vi "poly_range_DBL.vi"(8 "inclusive (T)":bool=TRUE, 9 "end":dbl, 10 "beginning":dbl) -> (1 "range":dbl[](array[numeric]), 2 "N":i32)   [LabVIEW 2015]
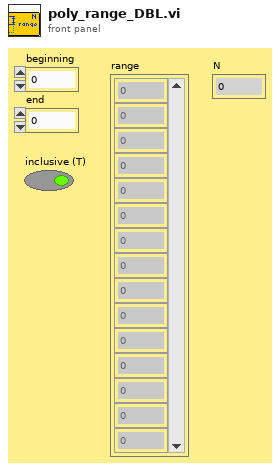
[diagram p1: front panel]
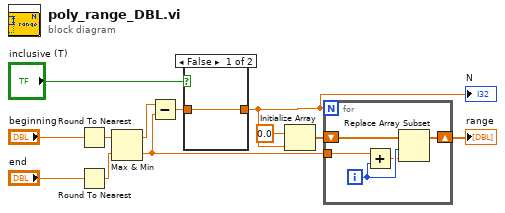
[diagram p0: block diagram]
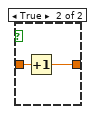
[diagram p2: hidden frame]
diagram:
  n1 = Round To Nearest(number="beginning") -> (nearest integer value=w3:dbl)
  n2 = Round To Nearest(number="end") -> (nearest integer value=w1:dbl)
  n3 = Max & Min(x=w3, y=w1) -> (max(x,y)=w12:dbl, min(x,y)=w9:dbl)
  n4 = Subtract(x=w12, y=w9) -> (x-y=w7:dbl)
  n5 = case shown="False" "inclusive (T)" {
    tunnel: w7 -> [w13 w15]
    tunnel: [w13 w14] -> w6
    frame False {
    }
    frame True {
      n6 = Increment(x=w15) -> (x+1=w14:dbl)
    }
  }
  "N" <- w6
  n7 = Initialize Array(0.0, w6) -> (w10:dbl[])
  n8 = for {
    N: w6 -> [_]
    shift-right: [w16] -> w8
    shift-left: w10 -> [w20]
    tunnel: w9 -> [w19]
    i -> [w18]
    n9 = Add(x=w19, y=w18) -> (x+y=w17:dbl)
    n10 = Replace Array Subset(array=w20, new element=w17, index=w18) -> (w16:dbl[])
  }
  "range" <- w8
